vi "Autonomous.vi"   [LabVIEW 2016]
doc: "This VI starts when autonomous period begins, and will automatically be terminated when it ends. You can carry out timed or sensor driven operations directly to I/O or to subsystems without needing to return to the caller."
uses:
  <vilib>/Rock Robotics/WPI/ThirdParty/CanMotor/TalonSRX/WPI_CANTalonSRX_BrakeOverride.ctl
  <vilib>/Rock Robotics/WPI/ThirdParty/CanMotor/TalonSRX/WPI_CANTalonSRX_APIControlMode.ctl
  <vilib>/Rock Robotics/WPI/Utilities/WPI_GetSetVariantRefNum.vi
  <vilib>/Rock Robotics/Network Tables/NT Read String.vi
  Framework/Robot Global Data.vi
  <vilib>/Rock Robotics/Network Tables/NT Read Number.vi
types:
  T1 = typedef "WPI_CANTalonSRX_BrakeOverride.ctl" = enum8{"No Override", "Override to Coast", "Override to Brake"}
  T2 = typedef "WPI_JoystickDevRef.ctl" = cluster{"Device":T3}
  T3 = typedef "WPI_JoystickDeviceEnum.ctl" = enum16{"USB 0", "USB 1", "USB 2", "USB 3", "USB 4", "USB 5"}
  T4 = typedef "WPI_RobotDriveDevRef.ctl" = cluster{"DevStatus":errorcluster, "Motors[]":T5[], "Square Inputs":bool, "Max Output":dbl}
  T5 = typedef "WPI_MotorControlDeviceRef.ctl" = cluster{"DeviceStatus":errorcluster, "Type":T6, "PWM":cluster{"PWM Channel":T7, "DeadBand":T8}, "CAN":cluster{"Device Number":u8, "SetOutput VI Ref":variant, "GetOutput VI Ref":variant, "Enable VI Ref":variant, "Disable VI Ref":variant, "Data":variant}, "Invert":bool}
  T6 = typedef "WPI_MotorControlType.ctl" = enum16{"PWM", "CAN"}
  T7 = typedef "FPGA_DIOPWMChannel.ctl" = enum8{"PWM 0", "PWM 1", "PWM 2", "PWM 3", "PWM 4", "PWM 5", "PWM 6", "PWM 7", "PWM 8", "PWM 9", "PWM MXP 0", "PWM MXP 1", "PWM MXP 2", "PWM MXP 3", "PWM MXP 4", "PWM MXP 5", "PWM MXP 6", "PWM MXP 7", "PWM MXP 8", "PWM MXP 9", "Invalid"}
  T8 = typedef "WPI_PWMDeadband.ctl" = cluster{"Name":string, "maxPositivePwm":i32, "minPositivePwm":i32, "centerPwm":i32, "maxNegativePwm":i32, "minNegativePwm":i32, "angularRange":u16}
  T9 = typedef "WPI_CANTalonSRX_APIControlMode.ctl" = enum8{"Percent VBus", "Speed", "Position", "Slave", "Unchanged / Invalid", "Voltage Compensation", "Current", "Motion Profile", "Motion Magic"}
  T10 = typedef "WPI_DigitalInputDevRef.ctl" = cluster{"DevStatus":errorcluster, "DIO Channel":T11}
  T11 = typedef "FPGA_DIOChannel.ctl" = enum8{"DIO 0", "DIO 1", "DIO 2", "DIO 3", "DIO 4", "DIO 5", "DIO 6", "DIO 7", "DIO 8", "DIO 9", "DIO MXP 0", "DIO MXP 1", "DIO MXP 2", "DIO MXP 3", "DIO MXP 4", "DIO MXP 5", "DIO MXP 6", "DIO MXP 7", "DIO MXP 8", "DIO MXP 9", "DIO MXP 10", "DIO MXP 11", "DIO MXP 12", "DIO MXP 13", "DIO MXP 14", "DIO MXP 15", "SPI Port CS1", "SPI Port CS2", "SPI Port CS3", "SPI Port MISO", "SPI Port MOSI", "Invalid"}
  T12 = typedef "WPI_CANTalonSRX_GlobalStatus.ctl" = cluster{"Applied Throttle":dbl, "Module Enabled":bool, "CAN Error":errorcluster, "Closed Loop Error":dbl, "Forward Limit Switch Closed":bool, "Reverse Limit Switch Closed":bool, "Sensor Position":dbl, "Sensor Velocity":dbl, "Current":dbl, "Sticky Fault - Over Temp":bool, "Sticky Fault - Under Voltage":bool, "Sticky Fault - Forward Limit":bool, "Sticky Fault - Reverse Limit":bool, "Sticky Fault - Forward Soft Limit":bool, "Sticky Fault - Reverse Soft Limit":bool, "Brake is Enabled":bool, "Encoder Position":dbl, "Encoder Velocity":dbl, "Encoder Index Count":dbl, "Encoder A Pin State":bool, "Encoder B Pin State":bool, "Encoder Index Pin State":bool, "Analog In":dbl, "Analog In Velocity":dbl, "Temperature (C)":dbl, "Battery Voltage":dbl, "Control 5 Is Supported":bool, "Current Profile Slot Select":dbl, "Pos Div 8":bool, "Vel Div 4":bool, "Pulse Width Position":i32, "Pulse Width Velocity":i32, "Pulse Width Rise To Rise (us)":i32, "Pulse Width Rise To Fall (us)":i32, "Mot Prof Active Is Under Run":bool, "Mot Prof Active Has Under Run":bool, "Mot Prof Active Is Last":bool, "Mot Prof Active Velocity Only":bool, "Mot Prof Active Is Valid":bool, "Mot Prof Buffer Is Full":bool, "Mot Prof Active Profile Slot Select":i32, "Mot Prof NextID":i32, "Mot Prof Count":i32, "Mot Prof Active Velocity":dbl, "Mot Prof Active Position":dbl, "Mot Prof Output Enable":i32}
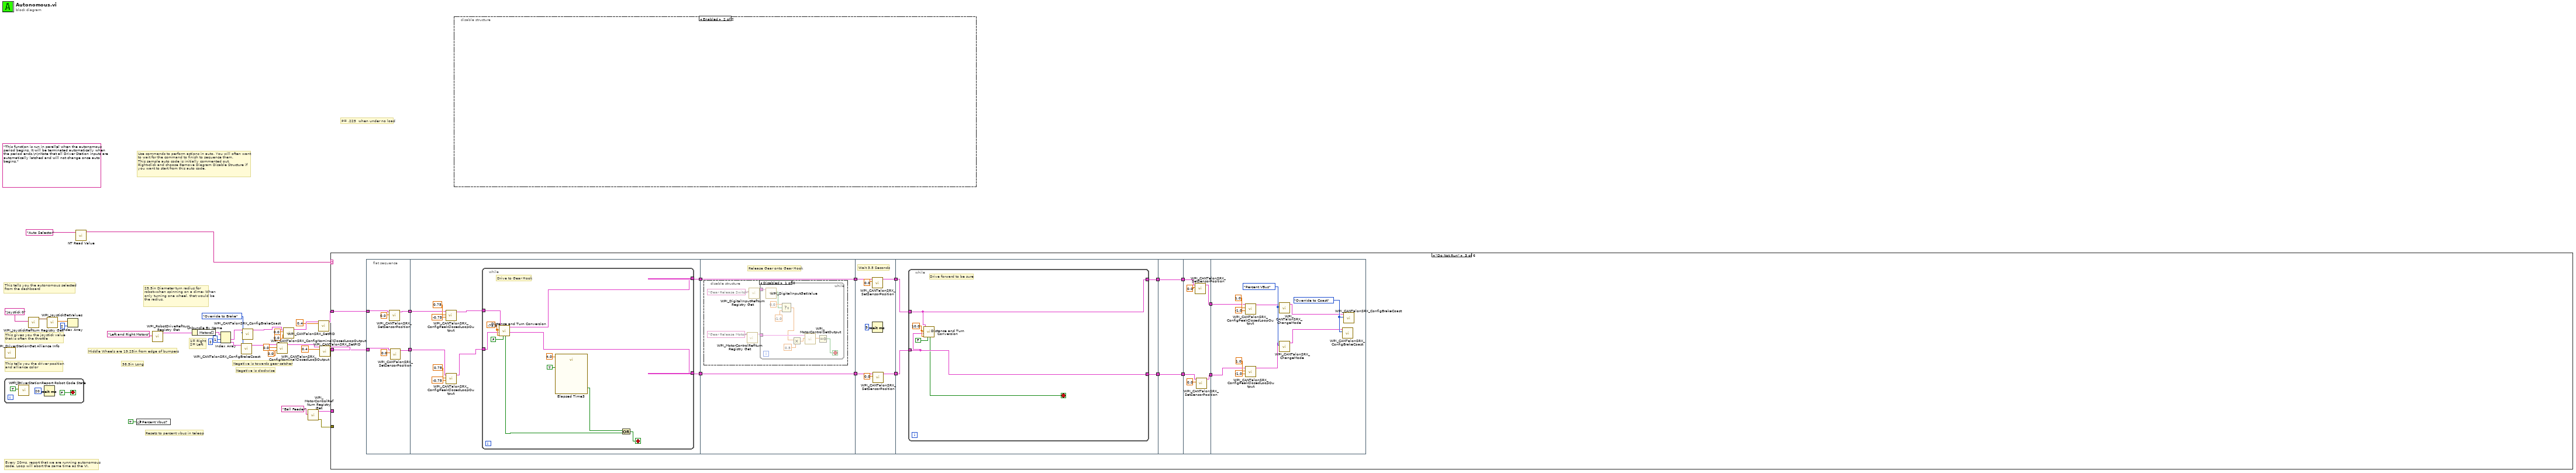
[diagram p0: block diagram]
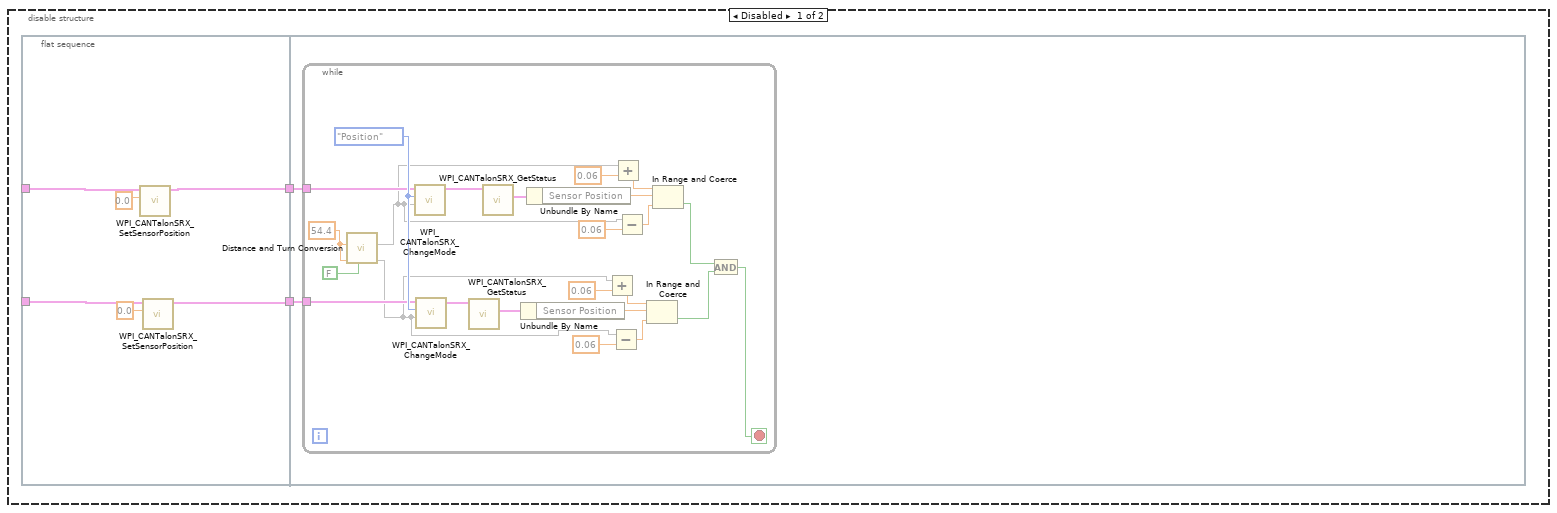
[diagram p2: hidden frame]
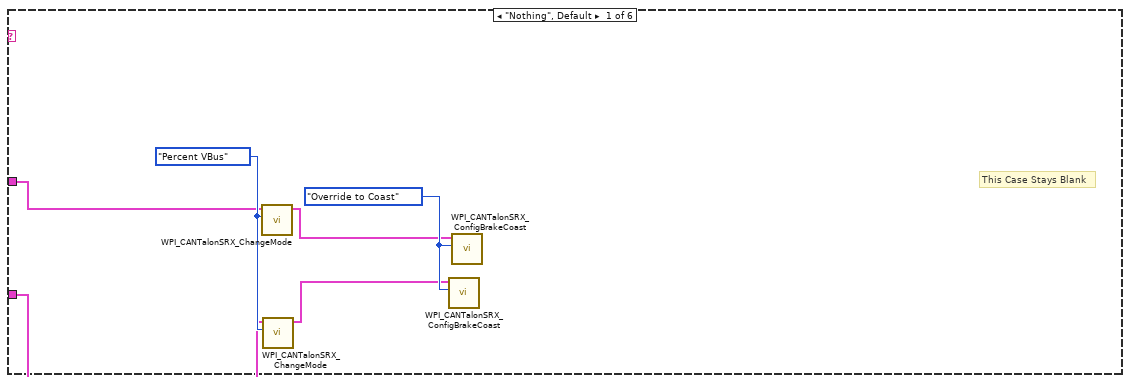
[diagram p3: hidden frame]
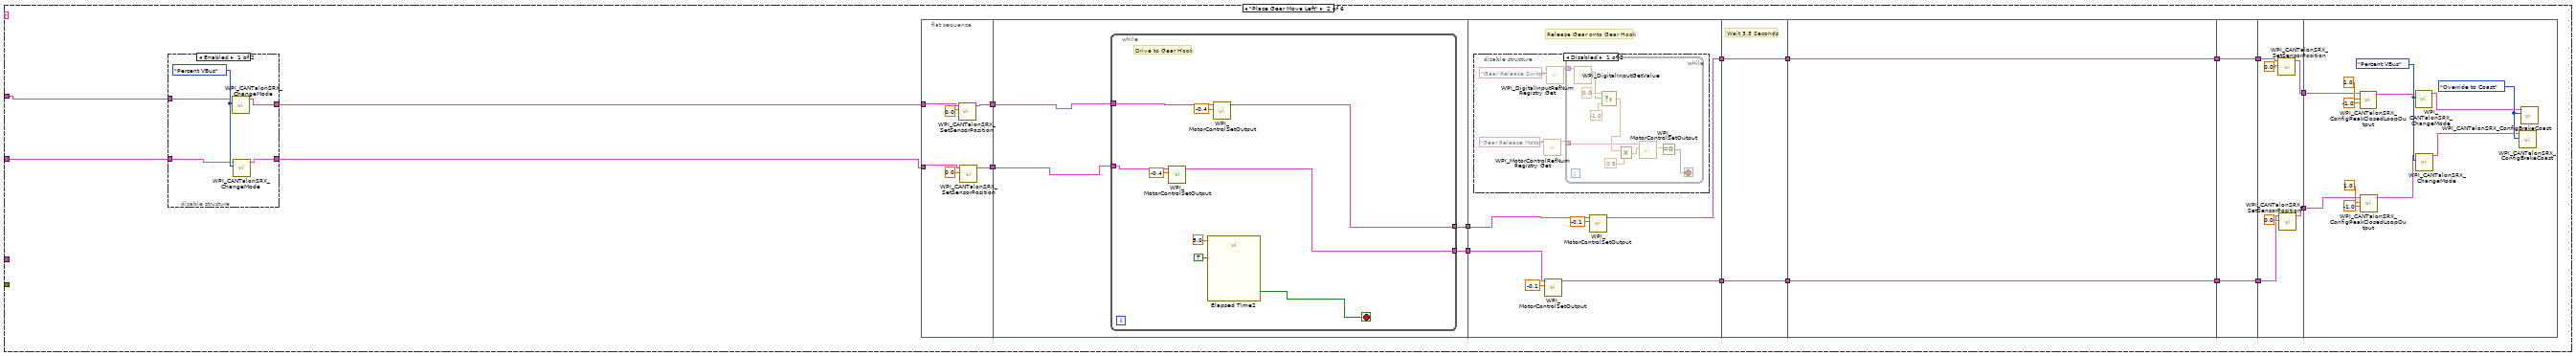
[diagram p4: hidden frame]
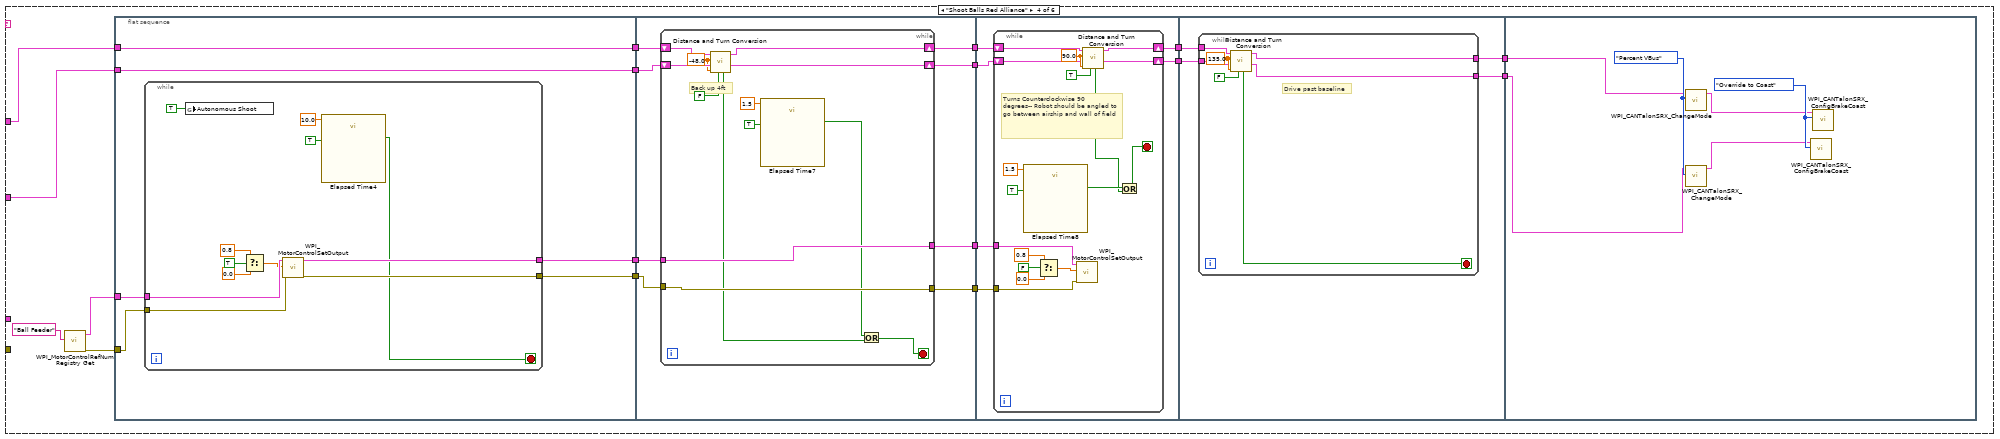
[diagram p8: hidden frame]
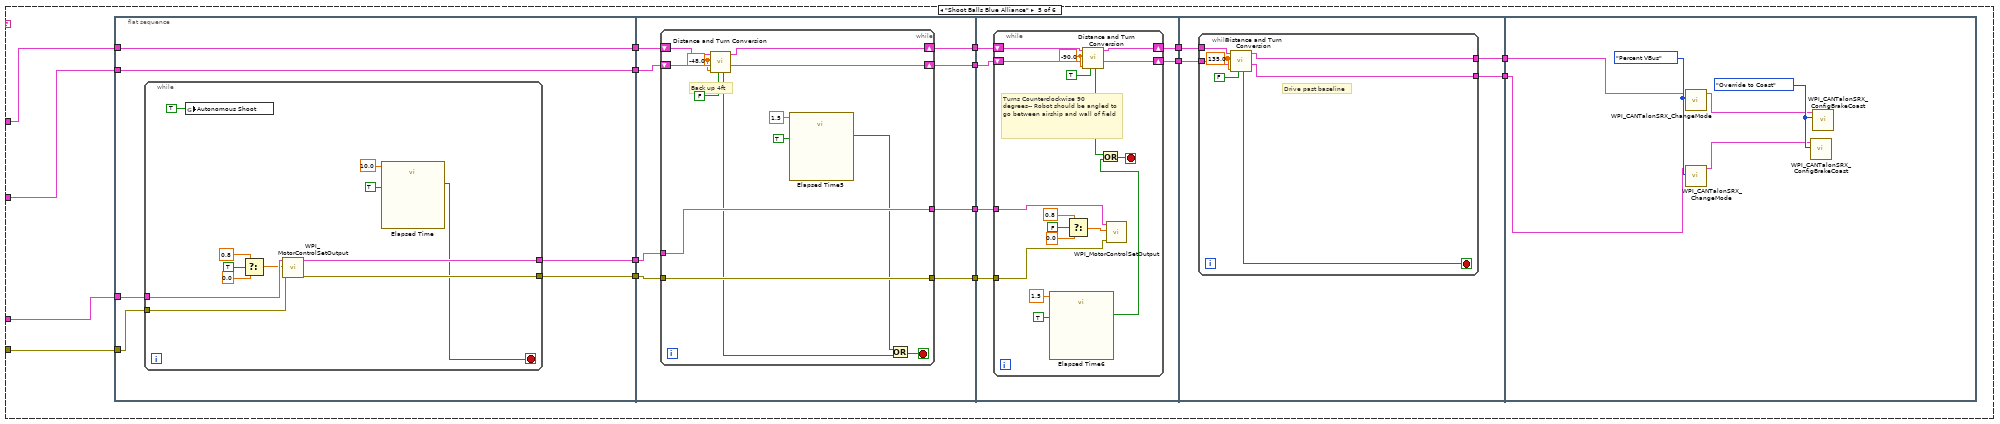
[diagram p9: hidden frame]
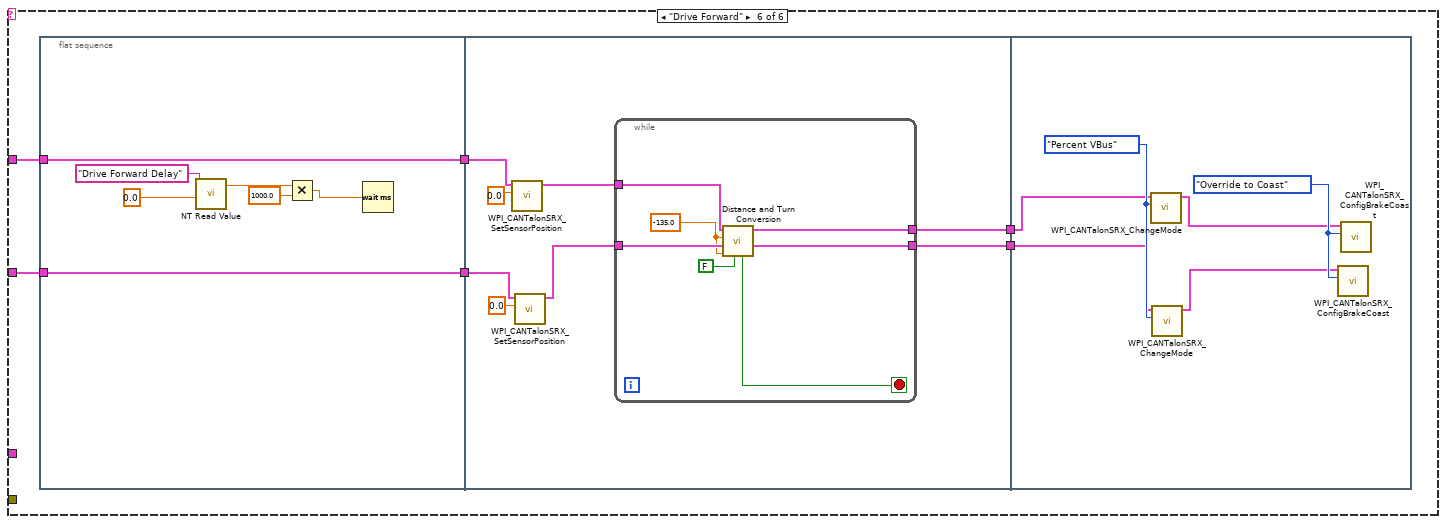
[diagram p10: hidden frame]
diagram:
  w14 = WPI_CANTalonSRX_BrakeOverride."Override to Brake" ("Brake / Coast Mode")
  (unwired) "This function is run in parallel when the autonomous period begins. It will be terminated automatically when the period ends.\n\nNote that all Driver Station inputs are automatically latched and will not change once auto begins."
  # "Negative is clockwise"
  # "Negative is towards gear catcher"
  # "Resets to percent vbus in teleop"
  # "38.5in Long"
  # "Middle Wheels are 19.25in from edge of bumpers"
  # "1= Right\n2= Left"
  # "25.5in Diameter turn radius for robot--when spinning on a dime- When only turning one wheel, that would be the radius."
  # "P= .225  when under no load"
  # "This tells you the autonomous selected\nfrom the dashboard"
  # "Every 20ms, report that we are running autonomous\ncode. Loop will abort the same time as the VI."
  # "This gives you the joystick value\nthat is often the throttle"
  # "Use commands to perform actions in auto. You will often want\nto wait for the command to finish to sequence them.\nThis sample auto code is initially commented out. \nRight-click and choose Remove Diagram Disable Structure if\nyou want to start from this auto code."
  # "This tells you the driver position\nand alliance color"
  n1 = while {
    stop <- FALSE stop-if-true
    n2 = call <vilib>:"WPI_DriverStationReport Robot Code State.vi"("Autonomous"=TRUE) -> ()  [unwired: 10 in, 1 out]
    n3 = Wait (ms)(milliseconds to wait=u32 20) -> ()  [unwired: 1 out]
  }
  n4 = call <vilib>:"WPI_DriverStationGet Alliance Info.vi"() -> ()  [unwired: 12 out]
  n5 = call <vilib>:"WPI_JoystickRefNum Registry Get.vi"("refnum name"="Joystick 0") -> ("JoystickDevRef"=w29:T2)  [unwired: 1 in, 9 out]
  n6 = call <vilib>:"WPI_JoystickGetValues.vi"("JoystickDevRef"=w29) -> ("Axes"=w28:dbl[])  [unwired: 6 in, 4 out]
  n7 = Index Array(array=w28, index=2) -> ()  [unwired: 1 out]
  n8 = call-poly <vilib>:"NT Read Value.vi"("Name"="Auto Selector") -> ("String"=w25:string)  [unwired: 9 in, 1 out]
  n9 = global write "Robot Global Data.vi" "Percent Vbus?"(TRUE ("Percent Vbus?")) -> ()
  n10 = call <vilib>:"WPI_RobotDriveRefNum Registry Get.vi"("refnum name"="Left and Right Motors") -> ("RobotDriveDevRef"=w19:T4)  [unwired: 9 in, 1 out]
  n11 = Unbundle By Name(w19) -> ("Motors[]"=w22:T5[])
  n12 = Index Array(array=w22, index #1=1 ("index"), index #2=2 ("index")) -> (element #1=w15:T5, element #2=w16:T5)
  n13 = call <vilib>:"WPI_CANTalonSRX_ConfigBrakeCoast.vi"("Brake / Coast Mode"=w14, "CAN Talon SRX Ref"=w16) -> ("CAN Talon SRX Ref"=w13:T5)  [unwired: 8 in, 1 out]
  n14 = call <vilib>:"WPI_CANTalonSRX_ConfigBrakeCoast.vi"("Brake / Coast Mode"=w14, "CAN Talon SRX Ref"=w15) -> ("CAN Talon SRX Ref"=w11:T5)  [unwired: 8 in, 1 out]
  n15 = call <vilib>:"WPI_CANTalonSRX_ConfigNominalClosedLoopOutput.vi"("Reverse Nominal Output"=0.0, "Forward Nominal Output"=0.0, "CAN Talon SRX Ref"=w13) -> ("CAN Talon SRX Ref"=w12:T5)  [unwired: 7 in, 1 out]
  n16 = call <vilib>:"WPI_CANTalonSRX_ConfigNominalClosedLoopOutput.vi"("Reverse Nominal Output"=0.0, "Forward Nominal Output"=0.0, "CAN Talon SRX Ref"=w11) -> ("CAN Talon SRX Ref"=w10:T5)  [unwired: 7 in, 1 out]
  n17 = call <vilib>:"WPI_MotorControlRefNum Registry Get.vi"("refnum name"="Ball Feeder") -> ("error out"=w1:errorcluster, "MotorControlDevRef"=w2:T5)  [unwired: 9 in]
  n18 = call <vilib>:"WPI_CANTalonSRX_SetPID.vi"("CAN Talon SRX Ref"=w10, "P"=0.4) -> ("CAN Talon SRX Ref"=w18:T5)  [unwired: 12 in, 1 out]
  n19 = call <vilib>:"WPI_CANTalonSRX_SetPID.vi"("CAN Talon SRX Ref"=w12, "P"=0.4) -> ("CAN Talon SRX Ref"=w17:T5)  [unwired: 12 in, 1 out]
  n20 = case shown="\"Do Not Run\"" w25 {
    tunnel: w18 -> [w35 w53 w143 w236 w334 w418]
    tunnel: w17 -> [w34 w51 w142 w235 w333 w419]
    tunnel: w2 -> [_ _ _ _ w322 _]
    tunnel: w1 -> [_ _ _ _ w321 _]
    frame "Nothing", Default {
      w38 = WPI_CANTalonSRX_BrakeOverride."Override to Coast" ("Brake / Coast Mode")
      w39 = WPI_CANTalonSRX_APIControlMode."Percent VBus" ("Control Mode")
      # "This Case Stays Blank"
      n21 = call <vilib>:"WPI_CANTalonSRX_ChangeMode.vi"("Control Mode"=w39, "CAN Talon SRX Ref"=w35) -> ("CAN Talon SRX Ref"=w37:T5)  [unwired: 8 in, 1 out]
      n22 = call <vilib>:"WPI_CANTalonSRX_ChangeMode.vi"("Control Mode"=w39, "CAN Talon SRX Ref"=w34) -> ("CAN Talon SRX Ref"=w36:T5)  [unwired: 8 in, 1 out]
      n23 = call <vilib>:"WPI_CANTalonSRX_ConfigBrakeCoast.vi"("Brake / Coast Mode"=w38, "CAN Talon SRX Ref"=w36) -> ()  [unwired: 8 in, 2 out]
      n24 = call <vilib>:"WPI_CANTalonSRX_ConfigBrakeCoast.vi"("Brake / Coast Mode"=w38, "CAN Talon SRX Ref"=w37) -> ()  [unwired: 8 in, 2 out]
    }
    frame "Place Gear Move Left" {
      n25 = disable-structure shown="Enabled" {
        disable-tunnel: w53 -> [w61 w64]
        disable-tunnel: [w60 w64] -> w52
        disable-tunnel: w51 -> [w59 w63]
        disable-tunnel: [w58 w63] -> w50
        frame Enabled {
          w62 = WPI_CANTalonSRX_APIControlMode."Percent VBus" ("Control Mode")
          n26 = call <vilib>:"WPI_CANTalonSRX_ChangeMode.vi"("Control Mode"=w62, "CAN Talon SRX Ref"=w61) -> ("CAN Talon SRX Ref"=w60:T5)  [unwired: 8 in, 1 out]
          n27 = call <vilib>:"WPI_CANTalonSRX_ChangeMode.vi"("Control Mode"=w62, "CAN Talon SRX Ref"=w59) -> ("CAN Talon SRX Ref"=w58:T5)  [unwired: 8 in, 1 out]
        }
        frame Disabled {
        }
      }
      n28 = flat-sequence {
        tunnel: w50 -> [w66]
        tunnel: w52 -> [w67]
        tunnel: [w65] -> w57
        tunnel: [w68] -> w56
        tunnel: w57 -> [w74]
        tunnel: w56 -> [w73]
        tunnel: [w72] -> w49
        tunnel: [w71] -> w48
        tunnel: w49 -> [w87]
        tunnel: w48 -> [w86]
        tunnel: [w85] -> w44
        tunnel: [w84] -> w43
        tunnel: [w105] -> w45
        tunnel: w44 -> [w105]
        tunnel: w43 -> [w104]
        tunnel: [w104] -> w42
        tunnel: [w107] -> w46
        tunnel: w45 -> [w107]
        tunnel: w42 -> [w106]
        tunnel: [w106] -> w41
        tunnel: [w109] -> w47
        tunnel: w46 -> [w109]
        tunnel: w41 -> [w108]
        tunnel: [w108] -> w40
        tunnel: [w113] -> w55
        tunnel: [w112] -> w54
        tunnel: w47 -> [w111]
        tunnel: w40 -> [w110]
        tunnel: w55 -> [w119]
        tunnel: w54 -> [w117]
        frame #0 {
          n29 = call <vilib>:"WPI_CANTalonSRX_SetSensorPosition.vi"("New Sensor Position"=0.0, "CAN Talon SRX Ref"=w67) -> ("CAN Talon SRX Ref"=w68:T5)  [unwired: 8 in, 1 out]
          n30 = call <vilib>:"WPI_CANTalonSRX_SetSensorPosition.vi"("New Sensor Position"=0.0, "CAN Talon SRX Ref"=w66) -> ("CAN Talon SRX Ref"=w65:T5)  [unwired: 8 in, 1 out]
        }
        frame #1 {
          n31 = while {
            tunnel: w73 -> [w81]
            tunnel: w74 -> [w80]
            tunnel: [w77] -> w72
            tunnel: [w76] -> w71
            stop <- w75 stop-if-true
            # "Drive to Gear Hook"
            n32 = call <vilib>:"WPI_MotorControlSetOutput.vi"("Output"=-0.4, "MotorControlDevRef"=w80) -> ("MotorControlDevRef"=w76:T5)  [unwired: 7 in, 2 out]
            n33 = call "Elapsed Time2"("Time Target (s)"=5.0, "Auto Reset"=TRUE) -> ("Time has Elapsed"=w75:bool)  [unwired: 10 in, 7 out]
            n34 = call <vilib>:"WPI_MotorControlSetOutput.vi"("Output"=-0.4, "MotorControlDevRef"=w81) -> ("MotorControlDevRef"=w77:T5)  [unwired: 7 in, 2 out]
          }
        }
        frame #2 {
          # "Release Gear onto Gear Hook"
          n35 = disable-structure shown="Disabled" {
            frame Disabled {
              n36 = call <vilib>:"WPI_MotorControlRefNum Registry Get.vi"("refnum name"="Gear Release Motor") -> ("MotorControlDevRef"=w90:T5)  [unwired: 9 in, 1 out]
              n37 = call <vilib>:"WPI_DigitalInputRefNum Registry Get.vi"("refnum name"="Gear Release Switch") -> ("DigitalInputDevRef"=w93:T10)  [unwired: 9 in, 1 out]
              n38 = while {
                tunnel: w93 -> [w103]
                tunnel: w90 -> [w102]
                stop <- w94 stop-if-true
                n39 = call <vilib>:"WPI_DigitalInputGetValue.vi"("DigitalInputDevRef"=w103) -> ("Value"=w96:bool)  [unwired: 8 in, 2 out]
                n40 = Select(t=0.0, s=w96, f=-1.0) -> (s? t:f=w98:dbl)
                n41 = Multiply(x=w98, y=0.5) -> (x*y=w100:dbl)
                n42 = call <vilib>:"WPI_MotorControlSetOutput.vi"("Output"=w100, "MotorControlDevRef"=w102) -> ("Motor Output"=w95:dbl)  [unwired: 7 in, 2 out]
                n43 = Equal To 0?(x=w95) -> (x = 0?=w94:bool)
              }
            }
            frame Enabled {
            }
          }
          n44 = call <vilib>:"WPI_MotorControlSetOutput.vi"("Output"=-0.1, "MotorControlDevRef"=w86) -> ("MotorControlDevRef"=w85:T5)  [unwired: 7 in, 2 out]
          n45 = call <vilib>:"WPI_MotorControlSetOutput.vi"("Output"=-0.1, "MotorControlDevRef"=w87) -> ("MotorControlDevRef"=w84:T5)  [unwired: 7 in, 2 out]
        }
        frame #3 {
          # "Wait 3.5 Seconds"
        }
        frame #4 {
        }
        frame #5 {
        }
        frame #6 {
          n46 = call <vilib>:"WPI_CANTalonSRX_SetSensorPosition.vi"("New Sensor Position"=0.0, "CAN Talon SRX Ref"=w110) -> ("CAN Talon SRX Ref"=w113:T5)  [unwired: 8 in, 1 out]
          n47 = call <vilib>:"WPI_CANTalonSRX_SetSensorPosition.vi"("New Sensor Position"=0.0, "CAN Talon SRX Ref"=w111) -> ("CAN Talon SRX Ref"=w112:T5)  [unwired: 8 in, 1 out]
        }
        frame #7 {
          w126 = WPI_CANTalonSRX_BrakeOverride."Override to Coast" ("Brake / Coast Mode")
          w127 = WPI_CANTalonSRX_APIControlMode."Percent VBus" ("Control Mode")
          n48 = call <vilib>:"WPI_CANTalonSRX_ConfigPeakClosedLoopOutput.vi"("Reverse Peak Output"=-1.0, "Forward Peak Output"=1.0, "CAN Talon SRX Ref"=w119) -> ("CAN Talon SRX Ref"=w118:T5)  [unwired: 7 in, 1 out]
          n49 = call <vilib>:"WPI_CANTalonSRX_ConfigPeakClosedLoopOutput.vi"("Reverse Peak Output"=-1.0, "Forward Peak Output"=1.0, "CAN Talon SRX Ref"=w117) -> ("CAN Talon SRX Ref"=w116:T5)  [unwired: 7 in, 1 out]
          n50 = call <vilib>:"WPI_CANTalonSRX_ChangeMode.vi"("Control Mode"=w127, "CAN Talon SRX Ref"=w118) -> ("CAN Talon SRX Ref"=w125:T5)  [unwired: 8 in, 1 out]
          n51 = call <vilib>:"WPI_CANTalonSRX_ChangeMode.vi"("Control Mode"=w127, "CAN Talon SRX Ref"=w116) -> ("CAN Talon SRX Ref"=w124:T5)  [unwired: 8 in, 1 out]
          n52 = call <vilib>:"WPI_CANTalonSRX_ConfigBrakeCoast.vi"("Brake / Coast Mode"=w126, "CAN Talon SRX Ref"=w124) -> ()  [unwired: 8 in, 2 out]
          n53 = call <vilib>:"WPI_CANTalonSRX_ConfigBrakeCoast.vi"("Brake / Coast Mode"=w126, "CAN Talon SRX Ref"=w125) -> ()  [unwired: 8 in, 2 out]
        }
      }
    }
    frame "Do Not Run" {
      n54 = flat-sequence {
        tunnel: w142 -> [w145]
        tunnel: w143 -> [w146]
        tunnel: [w144] -> w141
        tunnel: [w147] -> w140
        tunnel: w141 -> [w151]
        tunnel: w140 -> [w153]
        tunnel: [w159] -> w139
        tunnel: [w158] -> w138
        tunnel: w139 -> [w172]
        tunnel: w138 -> [w171]
        tunnel: [w172] -> w137
        tunnel: [w171] -> w136
        tunnel: w137 -> [w191]
        tunnel: w136 -> [w190]
        tunnel: [w189] -> w135
        tunnel: [w188] -> w134
        tunnel: w135 -> [w197]
        tunnel: w134 -> [w196]
        tunnel: [w195] -> w132
        tunnel: [w194] -> w129
        tunnel: [w204] -> w133
        tunnel: w132 -> [w204]
        tunnel: [w203] -> w130
        tunnel: w129 -> [w203]
        tunnel: w133 -> [w208]
        tunnel: [w207] -> w131
        tunnel: w130 -> [w206]
        tunnel: [w205] -> w128
        tunnel: w131 -> [w214]
        tunnel: w128 -> [w212]
        frame #0 {
          n55 = call <vilib>:"WPI_CANTalonSRX_SetSensorPosition.vi"("New Sensor Position"=0.0, "CAN Talon SRX Ref"=w146) -> ("CAN Talon SRX Ref"=w147:T5)  [unwired: 8 in, 1 out]
          n56 = call <vilib>:"WPI_CANTalonSRX_SetSensorPosition.vi"("New Sensor Position"=0.0, "CAN Talon SRX Ref"=w145) -> ("CAN Talon SRX Ref"=w144:T5)  [unwired: 8 in, 1 out]
        }
        frame #1 {
          n57 = call <vilib>:"WPI_CANTalonSRX_ConfigPeakClosedLoopOutput.vi"("Reverse Peak Output"=-0.75, "Forward Peak Output"=0.75, "CAN Talon SRX Ref"=w153) -> ("CAN Talon SRX Ref"=w152:T5)  [unwired: 7 in, 1 out]
          n58 = call <vilib>:"WPI_CANTalonSRX_ConfigPeakClosedLoopOutput.vi"("Reverse Peak Output"=-0.75, "Forward Peak Output"=0.75, "CAN Talon SRX Ref"=w151) -> ("CAN Talon SRX Ref"=w150:T5)  [unwired: 7 in, 1 out]
          n59 = while {
            tunnel: w152 -> [w168]
            tunnel: w150 -> [w167]
            tunnel: [w166] -> w159
            tunnel: [w165] -> w158
            stop <- w161 stop-if-true
            w170 = -75.0 ("Inches/Degrees Right")
            # "Drive to Gear Hook"
            n60 = call "Distance and Turn Conversion.vi"("Turn?"=FALSE, "Inches/Degrees Left"=w170, "CAN Talon SRX Ref Left In"=w167, "Inches/Degrees Right"=w170, "CAN Talon SRX Ref Right In"=w168) -> ("CAN Talon SRX Ref Left Out"=w165:T5, "CAN Talon SRX Ref Right Out"=w166:T5, "Both In Range"=w160:bool)  [unwired: 4 in]
            n61 = call "Elapsed Time3"("Time Target (s)"=4.0, "Auto Reset"=TRUE) -> ("Time has Elapsed"=w164:bool)  [unwired: 10 in, 7 out]
            n62 = Or(x=w164, y=w160) -> (x .or. y?=w161:bool)
          }
        }
        frame #2 {
          # "Release Gear onto Gear Hook"
          n63 = disable-structure shown="Disabled" {
            frame Disabled {
              n64 = call <vilib>:"WPI_MotorControlRefNum Registry Get.vi"("refnum name"="Gear Release Motor") -> ("MotorControlDevRef"=w173:T5)  [unwired: 9 in, 1 out]
              n65 = call <vilib>:"WPI_DigitalInputRefNum Registry Get.vi"("refnum name"="Gear Release Switch") -> ("DigitalInputDevRef"=w176:T10)  [unwired: 9 in, 1 out]
              n66 = while {
                tunnel: w176 -> [w186]
                tunnel: w173 -> [w185]
                stop <- w177 stop-if-true
                n67 = call <vilib>:"WPI_DigitalInputGetValue.vi"("DigitalInputDevRef"=w186) -> ("Value"=w179:bool)  [unwired: 8 in, 2 out]
                n68 = Select(t=0.0, s=w179, f=-1.0) -> (s? t:f=w181:dbl)
                n69 = Multiply(x=w181, y=0.5) -> (x*y=w183:dbl)
                n70 = call <vilib>:"WPI_MotorControlSetOutput.vi"("Output"=w183, "MotorControlDevRef"=w185) -> ("Motor Output"=w178:dbl)  [unwired: 7 in, 2 out]
                n71 = Equal To 0?(x=w178) -> (x = 0?=w177:bool)
              }
            }
            frame Enabled {
            }
          }
        }
        frame #3 {
          # "Wait 3.5 Seconds"
          n72 = Wait (ms)(milliseconds to wait=u32 9) -> ()  [unwired: 1 out]
          n73 = call <vilib>:"WPI_CANTalonSRX_SetSensorPosition.vi"("New Sensor Position"=0.0, "CAN Talon SRX Ref"=w191) -> ("CAN Talon SRX Ref"=w189:T5)  [unwired: 8 in, 1 out]
          n74 = call <vilib>:"WPI_CANTalonSRX_SetSensorPosition.vi"("New Sensor Position"=0.0, "CAN Talon SRX Ref"=w190) -> ("CAN Talon SRX Ref"=w188:T5)  [unwired: 8 in, 1 out]
        }
        frame #4 {
          n75 = while {
            tunnel: w197 -> [w200]
            tunnel: w196 -> [w199]
            tunnel: [w200] -> w195
            tunnel: [w199] -> w194
            stop <- w198 stop-if-true
            w202 = 10.0 ("Inches/Degrees Right")
            # "Drive forward to be sure"
            n76 = call "Distance and Turn Conversion.vi"("Turn?"=FALSE, "Inches/Degrees Left"=w202, "CAN Talon SRX Ref Left In"=w199, "Inches/Degrees Right"=w202, "CAN Talon SRX Ref Right In"=w200) -> ("Both In Range"=w198:bool)  [unwired: 4 in, 2 out]
          }
        }
        frame #5 {
        }
        frame #6 {
          n77 = call <vilib>:"WPI_CANTalonSRX_SetSensorPosition.vi"("New Sensor Position"=0.0, "CAN Talon SRX Ref"=w208) -> ("CAN Talon SRX Ref"=w207:T5)  [unwired: 8 in, 1 out]
          n78 = call <vilib>:"WPI_CANTalonSRX_SetSensorPosition.vi"("New Sensor Position"=0.0, "CAN Talon SRX Ref"=w206) -> ("CAN Talon SRX Ref"=w205:T5)  [unwired: 8 in, 1 out]
        }
        frame #7 {
          w221 = WPI_CANTalonSRX_BrakeOverride."Override to Coast" ("Brake / Coast Mode")
          w222 = WPI_CANTalonSRX_APIControlMode."Percent VBus" ("Control Mode")
          n79 = call <vilib>:"WPI_CANTalonSRX_ConfigPeakClosedLoopOutput.vi"("Reverse Peak Output"=-1.0, "Forward Peak Output"=1.0, "CAN Talon SRX Ref"=w214) -> ("CAN Talon SRX Ref"=w213:T5)  [unwired: 7 in, 1 out]
          n80 = call <vilib>:"WPI_CANTalonSRX_ConfigPeakClosedLoopOutput.vi"("Reverse Peak Output"=-1.0, "Forward Peak Output"=1.0, "CAN Talon SRX Ref"=w212) -> ("CAN Talon SRX Ref"=w211:T5)  [unwired: 7 in, 1 out]
          n81 = call <vilib>:"WPI_CANTalonSRX_ChangeMode.vi"("Control Mode"=w222, "CAN Talon SRX Ref"=w213) -> ("CAN Talon SRX Ref"=w220:T5)  [unwired: 8 in, 1 out]
          n82 = call <vilib>:"WPI_CANTalonSRX_ChangeMode.vi"("Control Mode"=w222, "CAN Talon SRX Ref"=w211) -> ("CAN Talon SRX Ref"=w219:T5)  [unwired: 8 in, 1 out]
          n83 = call <vilib>:"WPI_CANTalonSRX_ConfigBrakeCoast.vi"("Brake / Coast Mode"=w221, "CAN Talon SRX Ref"=w219) -> ()  [unwired: 8 in, 2 out]
          n84 = call <vilib>:"WPI_CANTalonSRX_ConfigBrakeCoast.vi"("Brake / Coast Mode"=w221, "CAN Talon SRX Ref"=w220) -> ()  [unwired: 8 in, 2 out]
        }
      }
    }
    frame "Shoot Balls Red Alliance" {
      n85 = call <vilib>:"WPI_MotorControlRefNum Registry Get.vi"("refnum name"="Ball Feeder") -> ("error out"=w237:errorcluster, "MotorControlDevRef"=w238:T5)  [unwired: 9 in]
      n86 = flat-sequence {
        tunnel: w235 -> [w244]
        tunnel: w236 -> [w245]
        tunnel: w237 -> [w242]
        tunnel: w238 -> [w243]
        tunnel: [w245] -> w230
        tunnel: [w244] -> w229
        tunnel: [w241] -> w228
        tunnel: [w240] -> w227
        tunnel: [w264] -> w234
        tunnel: [w263] -> w232
        tunnel: w230 -> [w265]
        tunnel: w229 -> [w262]
        tunnel: w228 -> [w260]
        tunnel: w227 -> [w259]
        tunnel: [w261] -> w224
        tunnel: [w258] -> w223
        tunnel: w234 -> [w284]
        tunnel: [w283] -> w233
        tunnel: w232 -> [w281]
        tunnel: [w282] -> w231
        tunnel: w224 -> [w280]
        tunnel: w223 -> [w279]
        tunnel: w233 -> [w305]
        tunnel: w231 -> [w304]
        tunnel: [w303] -> w226
        tunnel: [w302] -> w225
        tunnel: w226 -> [w314]
        tunnel: w225 -> [w313]
        frame #0 {
          n87 = while {
            tunnel: w243 -> [w256]
            tunnel: w242 -> [w255]
            tunnel: [w254] -> w241
            tunnel: [w253] -> w240
            stop <- w250 stop-if-true
            n88 = global write "Robot Global Data.vi" "Autonomous Shoot"(TRUE ("Percent Vbus?")) -> ()
            n89 = Select(t=0.8, s=TRUE, f=0.0) -> (s? t:f=w246:dbl)
            n90 = call <vilib>:"WPI_MotorControlSetOutput.vi"("error in (no error)"=w255, "Output"=w246, "MotorControlDevRef"=w256) -> ("error out"=w253:errorcluster, "MotorControlDevRef"=w254:T5)  [unwired: 6 in, 1 out]
            n91 = call "Elapsed Time4"("Time Target (s)"=10.0, "Auto Reset"=TRUE) -> ("Time has Elapsed"=w250:bool)  [unwired: 10 in, 7 out]
          }
        }
        frame #1 {
          n92 = while {
            shift-right: [w277] -> w264
            shift-left: w265 -> [w278]
            shift-right: [w276] -> w263
            shift-left: w262 -> [w275]
            tunnel: [w272] -> w261
            tunnel: w260 -> [w272]
            tunnel: w259 -> [w271]
            tunnel: [w271] -> w258
            stop <- w266 stop-if-true
            w274 = -48.0 ("Inches/Degrees Right")
            # "Back up 4ft"
            n93 = call "Distance and Turn Conversion.vi"("Turn?"=FALSE, "Inches/Degrees Left"=w274, "CAN Talon SRX Ref Left In"=w275, "Inches/Degrees Right"=w274, "CAN Talon SRX Ref Right In"=w278) -> ("CAN Talon SRX Ref Left Out"=w276:T5, "CAN Talon SRX Ref Right Out"=w277:T5, "Both In Range"=w267:bool)  [unwired: 4 in]
            n94 = call "Elapsed Time7"("Time Target (s)"=1.5, "Auto Reset"=TRUE) -> ("Time has Elapsed"=w268:bool)  [unwired: 10 in, 7 out]
            n95 = Or(x=w268, y=w267) -> (x .or. y?=w266:bool)
          }
        }
        frame #2 {
          n96 = while {
            shift-right: [w299] -> w283
            shift-left: w284 -> [w300]
            shift-right: [w298] -> w282
            shift-left: w281 -> [w297]
            tunnel: w280 -> [w291]
            tunnel: w279 -> [w290]
            stop <- w285 stop-if-true
            w301 = 90.0 ("Inches/Degrees Right")
            # "Turns Counterclockwise 90 degrees-- Robot should be angled to go between airship and wall of field"
            n97 = call "Elapsed Time8"("Time Target (s)"=1.5, "Auto Reset"=TRUE) -> ("Time has Elapsed"=w287:bool)  [unwired: 10 in, 7 out]
            n98 = Select(t=0.8, s=FALSE, f=0.0) -> (s? t:f=w292:dbl)
            n99 = call <vilib>:"WPI_MotorControlSetOutput.vi"("error in (no error)"=w290, "Output"=w292, "MotorControlDevRef"=w291) -> ()  [unwired: 6 in, 3 out]
            n100 = call "Distance and Turn Conversion.vi"("Turn?"=TRUE, "Inches/Degrees Left"=w301, "CAN Talon SRX Ref Left In"=w297, "Inches/Degrees Right"=w301, "CAN Talon SRX Ref Right In"=w300) -> ("CAN Talon SRX Ref Left Out"=w298:T5, "CAN Talon SRX Ref Right Out"=w299:T5, "Both In Range"=w286:bool)  [unwired: 4 in]
            n101 = Or(x=w287, y=w286) -> (x .or. y?=w285:bool)
          }
        }
        frame #3 {
          n102 = while {
            tunnel: w305 -> [w311]
            tunnel: w304 -> [w310]
            tunnel: [w307] -> w303
            tunnel: [w306] -> w302
            stop <- w309 stop-if-true
            w312 = 135.0 ("Inches/Degrees Right")
            # "Drive past baseline"
            n103 = call "Distance and Turn Conversion.vi"("Turn?"=FALSE, "Inches/Degrees Left"=w312, "CAN Talon SRX Ref Left In"=w310, "Inches/Degrees Right"=w312, "CAN Talon SRX Ref Right In"=w311) -> ("CAN Talon SRX Ref Left Out"=w306:T5, "CAN Talon SRX Ref Right Out"=w307:T5, "Both In Range"=w309:bool)  [unwired: 4 in]
          }
        }
        frame #4 {
          w317 = WPI_CANTalonSRX_BrakeOverride."Override to Coast" ("Brake / Coast Mode")
          w318 = WPI_CANTalonSRX_APIControlMode."Percent VBus" ("Control Mode")
          n104 = call <vilib>:"WPI_CANTalonSRX_ChangeMode.vi"("Control Mode"=w318, "CAN Talon SRX Ref"=w314) -> ("CAN Talon SRX Ref"=w316:T5)  [unwired: 8 in, 1 out]
          n105 = call <vilib>:"WPI_CANTalonSRX_ChangeMode.vi"("Control Mode"=w318, "CAN Talon SRX Ref"=w313) -> ("CAN Talon SRX Ref"=w315:T5)  [unwired: 8 in, 1 out]
          n106 = call <vilib>:"WPI_CANTalonSRX_ConfigBrakeCoast.vi"("Brake / Coast Mode"=w317, "CAN Talon SRX Ref"=w315) -> ()  [unwired: 8 in, 2 out]
          n107 = call <vilib>:"WPI_CANTalonSRX_ConfigBrakeCoast.vi"("Brake / Coast Mode"=w317, "CAN Talon SRX Ref"=w316) -> ()  [unwired: 8 in, 2 out]
        }
      }
    }
    frame "Shoot Balls Blue Alliance" {
      n108 = flat-sequence {
        tunnel: w333 -> [w339]
        tunnel: w334 -> [w340]
        tunnel: w321 -> [w337]
        tunnel: w322 -> [w338]
        tunnel: [w340] -> w328
        tunnel: [w339] -> w327
        tunnel: [w336] -> w326
        tunnel: [w335] -> w325
        tunnel: [w359] -> w332
        tunnel: [w358] -> w330
        tunnel: w328 -> [w360]
        tunnel: w327 -> [w357]
        tunnel: w326 -> [w356]
        tunnel: w325 -> [w354]
        tunnel: [w355] -> w320
        tunnel: [w353] -> w319
        tunnel: w332 -> [w379]
        tunnel: [w378] -> w331
        tunnel: w330 -> [w376]
        tunnel: [w377] -> w329
        tunnel: w320 -> [w375]
        tunnel: w319 -> [w374]
        tunnel: w331 -> [w400]
        tunnel: w329 -> [w399]
        tunnel: [w398] -> w324
        tunnel: [w397] -> w323
        tunnel: w324 -> [w409]
        tunnel: w323 -> [w408]
        frame #0 {
          n109 = while {
            tunnel: w338 -> [w349]
            tunnel: w337 -> [w348]
            tunnel: [w346] -> w336
            tunnel: [w345] -> w335
            stop <- w342 stop-if-true
            n110 = global write "Robot Global Data.vi" "Autonomous Shoot"(TRUE ("Percent Vbus?")) -> ()
            n111 = Select(t=0.8, s=TRUE, f=0.0) -> (s? t:f=w347:dbl)
            n112 = call <vilib>:"WPI_MotorControlSetOutput.vi"("error in (no error)"=w348, "Output"=w347, "MotorControlDevRef"=w349) -> ("error out"=w345:errorcluster, "MotorControlDevRef"=w346:T5)  [unwired: 6 in, 1 out]
            n113 = call "Elapsed Time"("Time Target (s)"=10.0, "Auto Reset"=TRUE) -> ("Time has Elapsed"=w342:bool)  [unwired: 10 in, 7 out]
          }
        }
        frame #1 {
          n114 = while {
            shift-right: [w372] -> w359
            shift-left: w360 -> [w373]
            shift-right: [w371] -> w358
            shift-left: w357 -> [w370]
            tunnel: w356 -> [w367]
            tunnel: [w367] -> w355
            tunnel: w354 -> [w366]
            tunnel: [w366] -> w353
            stop <- w362 stop-if-true
            w369 = -48.0 ("Inches/Degrees Right")
            # "Back up 4ft"
            n115 = call "Distance and Turn Conversion.vi"("Turn?"=FALSE, "Inches/Degrees Left"=w369, "CAN Talon SRX Ref Left In"=w370, "Inches/Degrees Right"=w369, "CAN Talon SRX Ref Right In"=w373) -> ("CAN Talon SRX Ref Left Out"=w371:T5, "CAN Talon SRX Ref Right Out"=w372:T5, "Both In Range"=w363:bool)  [unwired: 4 in]
            n116 = call "Elapsed Time5"("Time Target (s)"=1.5, "Auto Reset"=TRUE) -> ("Time has Elapsed"=w361:bool)  [unwired: 10 in, 7 out]
            n117 = Or(x=w361, y=w363) -> (x .or. y?=w362:bool)
          }
        }
        frame #2 {
          n118 = while {
            shift-right: [w394] -> w378
            shift-left: w379 -> [w395]
            shift-right: [w393] -> w377
            shift-left: w376 -> [w392]
            tunnel: w375 -> [w386]
            tunnel: w374 -> [w385]
            stop <- w382 stop-if-true
            w396 = -90.0 ("Inches/Degrees Right")
            # "Turns Counterclockwise 90 degrees-- Robot should be angled to go between airship and wall of field"
            n119 = call "Elapsed Time6"("Time Target (s)"=1.5, "Auto Reset"=TRUE) -> ("Time has Elapsed"=w380:bool)  [unwired: 10 in, 7 out]
            n120 = Select(t=0.8, s=FALSE, f=0.0) -> (s? t:f=w387:dbl)
            n121 = call "Distance and Turn Conversion.vi"("Turn?"=TRUE, "Inches/Degrees Left"=w396, "CAN Talon SRX Ref Left In"=w392, "Inches/Degrees Right"=w396, "CAN Talon SRX Ref Right In"=w395) -> ("CAN Talon SRX Ref Left Out"=w393:T5, "CAN Talon SRX Ref Right Out"=w394:T5, "Both In Range"=w381:bool)  [unwired: 4 in]
            n122 = Or(x=w381, y=w380) -> (x .or. y?=w382:bool)
            n123 = call <vilib>:"WPI_MotorControlSetOutput.vi"("error in (no error)"=w385, "Output"=w387, "MotorControlDevRef"=w386) -> ()  [unwired: 6 in, 3 out]
          }
        }
        frame #3 {
          n124 = while {
            tunnel: w400 -> [w406]
            tunnel: w399 -> [w405]
            tunnel: [w402] -> w398
            tunnel: [w401] -> w397
            stop <- w404 stop-if-true
            w407 = 135.0 ("Inches/Degrees Right")
            # "Drive past baseline"
            n125 = call "Distance and Turn Conversion.vi"("Turn?"=FALSE, "Inches/Degrees Left"=w407, "CAN Talon SRX Ref Left In"=w405, "Inches/Degrees Right"=w407, "CAN Talon SRX Ref Right In"=w406) -> ("CAN Talon SRX Ref Left Out"=w401:T5, "CAN Talon SRX Ref Right Out"=w402:T5, "Both In Range"=w404:bool)  [unwired: 4 in]
          }
        }
        frame #4 {
          w412 = WPI_CANTalonSRX_BrakeOverride."Override to Coast" ("Brake / Coast Mode")
          w413 = WPI_CANTalonSRX_APIControlMode."Percent VBus" ("Control Mode")
          n126 = call <vilib>:"WPI_CANTalonSRX_ChangeMode.vi"("Control Mode"=w413, "CAN Talon SRX Ref"=w409) -> ("CAN Talon SRX Ref"=w411:T5)  [unwired: 8 in, 1 out]
          n127 = call <vilib>:"WPI_CANTalonSRX_ChangeMode.vi"("Control Mode"=w413, "CAN Talon SRX Ref"=w408) -> ("CAN Talon SRX Ref"=w410:T5)  [unwired: 8 in, 1 out]
          n128 = call <vilib>:"WPI_CANTalonSRX_ConfigBrakeCoast.vi"("Brake / Coast Mode"=w412, "CAN Talon SRX Ref"=w410) -> ()  [unwired: 8 in, 2 out]
          n129 = call <vilib>:"WPI_CANTalonSRX_ConfigBrakeCoast.vi"("Brake / Coast Mode"=w412, "CAN Talon SRX Ref"=w411) -> ()  [unwired: 8 in, 2 out]
        }
      }
    }
    frame "Drive Forward" {
      n130 = flat-sequence {
        tunnel: w418 -> [w425]
        tunnel: w419 -> [w426]
        tunnel: [w426] -> w415
        tunnel: [w425] -> w414
        tunnel: [w428] -> w417
        tunnel: [w427] -> w416
        tunnel: w415 -> [w432]
        tunnel: w414 -> [w431]
        tunnel: w417 -> [w443]
        tunnel: w416 -> [w442]
        frame #0 {
          n131 = call-poly <vilib>:"NT Read Value.vi"("Default Value"=0.0, "Name"="Drive Forward Delay") -> ("Numeric"=w422:dbl)  [unwired: 8 in, 1 out]
          n132 = Multiply(x=w422, y=1000.0) -> (x*y=w420:dbl)
          n133 = Wait (ms)(milliseconds to wait=w420) -> ()  [unwired: 1 out]
        }
        frame #1 {
          n134 = call <vilib>:"WPI_CANTalonSRX_SetSensorPosition.vi"("New Sensor Position"=0.0, "CAN Talon SRX Ref"=w431) -> ("CAN Talon SRX Ref"=w430:T5)  [unwired: 8 in, 1 out]
          n135 = call <vilib>:"WPI_CANTalonSRX_SetSensorPosition.vi"("New Sensor Position"=0.0, "CAN Talon SRX Ref"=w432) -> ("CAN Talon SRX Ref"=w429:T5)  [unwired: 8 in, 1 out]
          n136 = while {
            tunnel: w430 -> [w440]
            tunnel: w429 -> [w439]
            tunnel: [w436] -> w428
            tunnel: [w435] -> w427
            stop <- w437 stop-if-true
            w438 = -135.0 ("Inches/Degrees Right")
            n137 = call "Distance and Turn Conversion.vi"("Turn?"=FALSE, "Inches/Degrees Left"=w438, "CAN Talon SRX Ref Left In"=w439, "Inches/Degrees Right"=w438, "CAN Talon SRX Ref Right In"=w440) -> ("CAN Talon SRX Ref Left Out"=w435:T5, "CAN Talon SRX Ref Right Out"=w436:T5, "Both In Range"=w437:bool)  [unwired: 4 in]
          }
        }
        frame #2 {
          w446 = WPI_CANTalonSRX_BrakeOverride."Override to Coast" ("Brake / Coast Mode")
          w447 = WPI_CANTalonSRX_APIControlMode."Percent VBus" ("Control Mode")
          n138 = call <vilib>:"WPI_CANTalonSRX_ChangeMode.vi"("Control Mode"=w447, "CAN Talon SRX Ref"=w443) -> ("CAN Talon SRX Ref"=w445:T5)  [unwired: 8 in, 1 out]
          n139 = call <vilib>:"WPI_CANTalonSRX_ChangeMode.vi"("Control Mode"=w447, "CAN Talon SRX Ref"=w442) -> ("CAN Talon SRX Ref"=w444:T5)  [unwired: 8 in, 1 out]
          n140 = call <vilib>:"WPI_CANTalonSRX_ConfigBrakeCoast.vi"("Brake / Coast Mode"=w446, "CAN Talon SRX Ref"=w444) -> ()  [unwired: 8 in, 2 out]
          n141 = call <vilib>:"WPI_CANTalonSRX_ConfigBrakeCoast.vi"("Brake / Coast Mode"=w446, "CAN Talon SRX Ref"=w445) -> ()  [unwired: 8 in, 2 out]
        }
      }
    }
  }
  n142 = disable-structure shown="Enabled" {
    frame Disabled {
      n143 = flat-sequence {
        tunnel: _ -> [w451]
        tunnel: _ -> [w452]
        tunnel: [w450] -> w449
        tunnel: [w453] -> w448
        tunnel: w449 -> [w456]
        tunnel: w448 -> [w457]
        frame #0 {
          n144 = call <vilib>:"WPI_CANTalonSRX_SetSensorPosition.vi"("New Sensor Position"=0.0, "CAN Talon SRX Ref"=w452) -> ("CAN Talon SRX Ref"=w453:T5)  [unwired: 8 in, 1 out]
          n145 = call <vilib>:"WPI_CANTalonSRX_SetSensorPosition.vi"("New Sensor Position"=0.0, "CAN Talon SRX Ref"=w451) -> ("CAN Talon SRX Ref"=w450:T5)  [unwired: 8 in, 1 out]
        }
        frame #1 {
          n146 = while {
            tunnel: w457 -> [w479]
            tunnel: w456 -> [w478]
            stop <- w460 stop-if-true
            w475 = 54.4 ("Inches/Degrees Right")
            w480 = WPI_CANTalonSRX_APIControlMode."Position" ("Control Mode")
            n147 = call "Distance and Turn Conversion.vi"("Turn?"=FALSE, "Inches/Degrees Left"=w475, "Inches/Degrees Right"=w475) -> (0:w461, 2:w469)  [unwired: 4 in, 3 out]
            n148 = call <vilib>:"WPI_CANTalonSRX_ChangeMode.vi"("Output"=w469, "Control Mode"=w480, "CAN Talon SRX Ref"=w479) -> ("CAN Talon SRX Ref"=w477:T5)  [unwired: 7 in, 1 out]
            n149 = call <vilib>:"WPI_CANTalonSRX_ChangeMode.vi"("Output"=w461, "Control Mode"=w480, "CAN Talon SRX Ref"=w478) -> ("CAN Talon SRX Ref"=w476:T5)  [unwired: 7 in, 1 out]
            n150 = call <vilib>:"WPI_CANTalonSRX_GetStatus.vi"("CAN Talon SRX Ref"=w476) -> ("Talon SRX Status"=w462:T12)  [unwired: 8 in, 2 out]
            n151 = call <vilib>:"WPI_CANTalonSRX_GetStatus.vi"("CAN Talon SRX Ref"=w477) -> ("Talon SRX Status"=w481:T12)  [unwired: 8 in, 2 out]
            n152 = Unbundle By Name(w462) -> ("Sensor Position"=w467:dbl)
            n153 = Unbundle By Name(w481) -> ("Sensor Position"=w473:dbl)
            n154 = Add(x=w461, y=0.06) -> (x+y=w466:dbl)
            n155 = Subtract(x=w461, y=0.06) -> (x-y=w464:dbl)
            n156 = Add(x=w469, y=0.06) -> (x+y=w472:dbl)
            n157 = Subtract(x=w469, y=0.06) -> (x-y=w470:dbl)
            n158 = In Range and Coerce(upper limit=w466, x=w467, lower limit=w464) -> (In Range?=w458:bool)  [unwired: 1 out]
            n159 = In Range and Coerce(upper limit=w472, x=w473, lower limit=w470) -> (In Range?=w459:bool)  [unwired: 1 out]
            n160 = And(x=w459, y=w458) -> (x .and. y?=w460:bool)
          }
        }
      }
    }
    frame Enabled {
    }
  }
